vi "view system reservations.vi"(10 "Variant":variant) -> ()   [LabVIEW 2016, in "FPGA Addon System Explorer.lvlib"]
uses:
  FPGA Addon System Explorer.lvlib
  <vilib>/NI VeriStand/Custom Device API/Custom Device API.lvlib
panel:
  in  "Tree":string(tree)
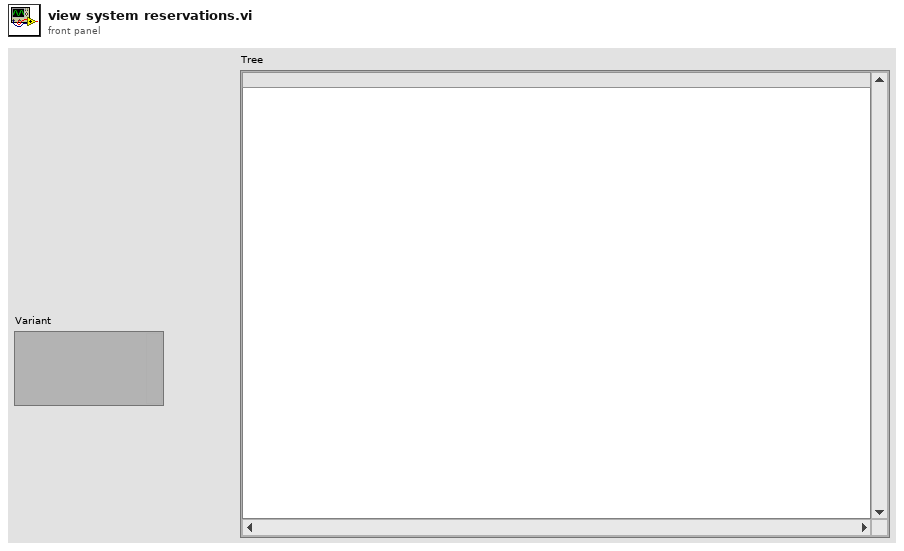
[diagram p1: front panel]
types:
  T1 = typedef "Custom Device API.lvlib/Custom Device Item Info.ctl" = cluster{"Name":string, "Is Channel":bool, "GUID":string, "Is Waveform":bool}
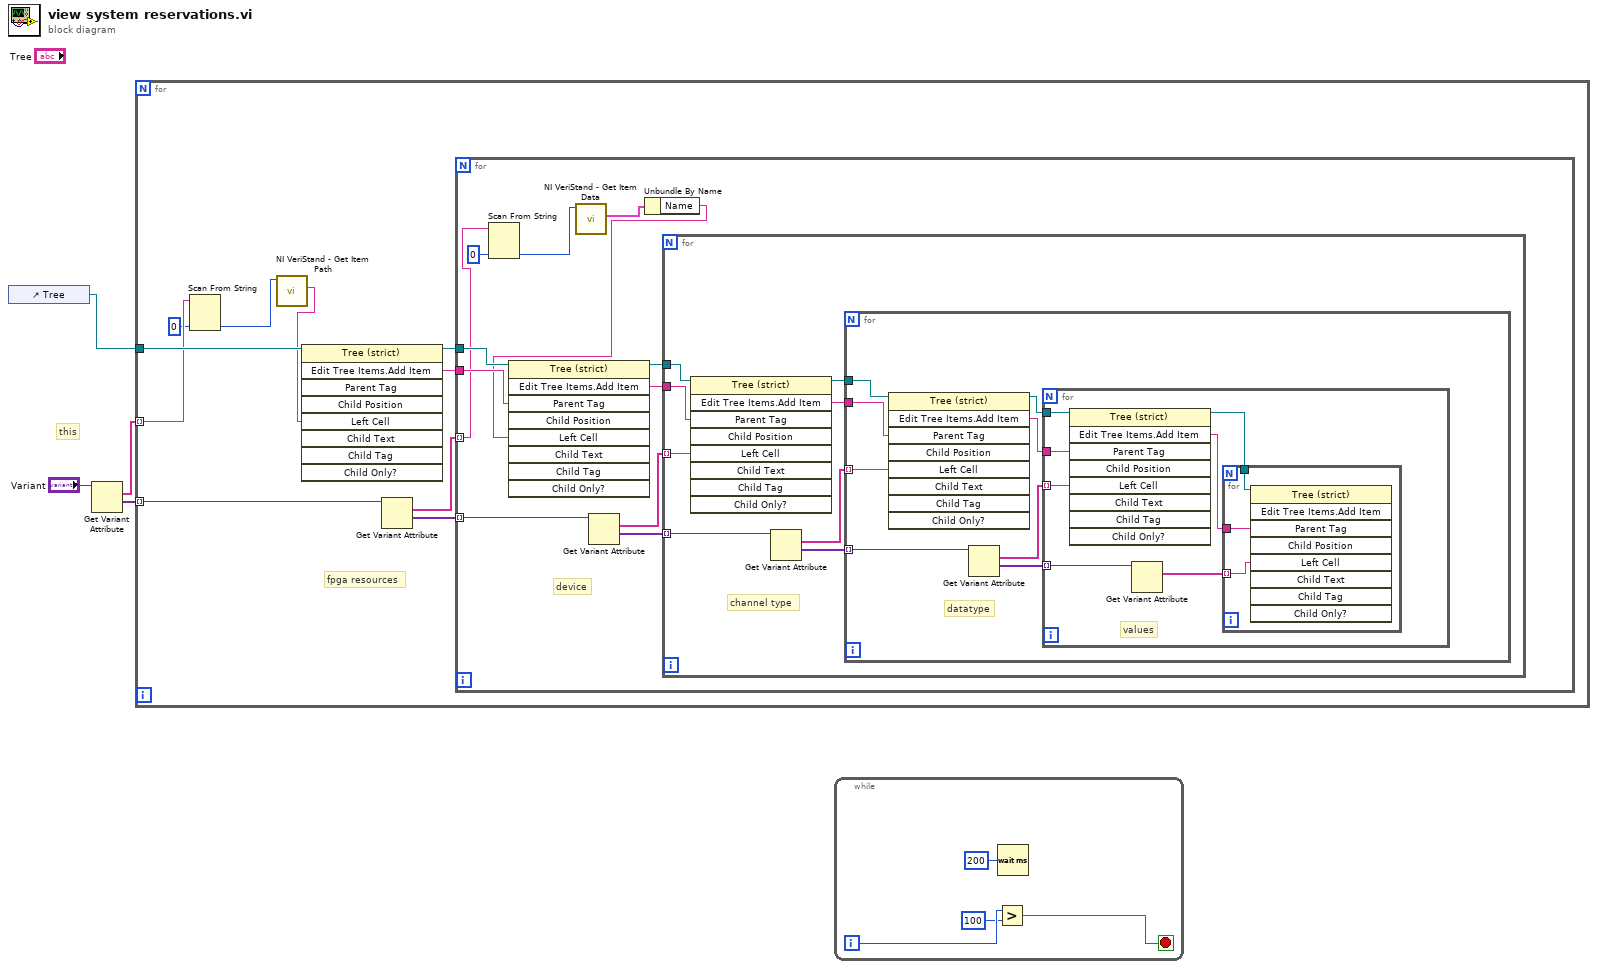
[diagram p0: block diagram]
diagram:
  # "this"
  n1 = control-ref of="Tree"() -> (w1:refnum<vi>)
  n2 = Get Variant Attribute(Variant="Variant") -> (names=w3:string[], values=w2:variant[])  [unwired: 3 in, 2 out]
  n3 = for {
    tunnel: w3 -> [w8] mode=indexing
    tunnel: w2 -> [w14] mode=indexing
    tunnel: w1 -> [w10]
    # "fpga resources"
    n4 = Scan From String(input string=w8, default 1=u64 0 ("default value 1")) -> (output 1=w6:u64)  [unwired: 3 in, 3 out]
    n5 = call <vilib>:"NI VeriStand - Get Item Path.vi"("Item Ref in"=w6) -> ("Path"=w5:string)  [unwired: 7 in, 3 out]
    n6 = invoke on="Invoke Node" class="Tree (strict)" method="Edit Tree Items.Add Item"(reference=w10, "Left Cell"=w5) -> (reference out=w9:refnum<vi>, "Edit Tree Items:Add Item"=w12:string)  [unwired: 7 in, 7 out]
    n7 = Get Variant Attribute(Variant=w14) -> (names=w13:string[], values=w11:variant[])  [unwired: 3 in, 2 out]
    n8 = for {
      tunnel: w13 -> [w15] mode=indexing
      tunnel: w12 -> [w26]
      tunnel: w11 -> [w24] mode=indexing
      tunnel: w9 -> [w21]
      # "device"
      n9 = Scan From String(input string=w15, default 1=u64 0 ("default value 1")) -> (output 1=w19:u64)  [unwired: 3 in, 3 out]
      n10 = call <vilib>:"NI VeriStand - Get Item Data.vi"("Item Ref in"=w19) -> ("Item Info"=w17:T1)  [unwired: 7 in, 3 out]
      n11 = Get Variant Attribute(Variant=w24) -> (names=w23:string[], values=w22:variant[])  [unwired: 3 in, 2 out]
      n12 = Unbundle By Name(w17) -> ("Name"=w16:string)
      n13 = invoke on="Invoke Node" class="Tree (strict)" method="Edit Tree Items.Add Item"(reference=w21, "Parent Tag"=w26, "Left Cell"=w16) -> (reference out=w20:refnum<vi>, "Edit Tree Items:Add Item"=w25:string)  [unwired: 6 in, 7 out]
      n14 = for {
        tunnel: w23 -> [w33] mode=indexing
        tunnel: w25 -> [w34]
        tunnel: w22 -> [w32] mode=indexing
        tunnel: w20 -> [w28]
        # "channel type"
        n15 = invoke on="Invoke Node" class="Tree (strict)" method="Edit Tree Items.Add Item"(reference=w28, "Parent Tag"=w34, "Left Cell"=w33) -> (reference out=w27:refnum<vi>, "Edit Tree Items:Add Item"=w30:string)  [unwired: 6 in, 7 out]
        n16 = Get Variant Attribute(Variant=w32) -> (names=w31:string[], values=w29:variant[])  [unwired: 3 in, 2 out]
        n17 = for {
          tunnel: w31 -> [w41] mode=indexing
          tunnel: w30 -> [w42]
          tunnel: w29 -> [w39] mode=indexing
          tunnel: w27 -> [w35]
          # "datatype"
          n18 = invoke on="Invoke Node" class="Tree (strict)" method="Edit Tree Items.Add Item"(reference=w35, "Parent Tag"=w42, "Left Cell"=w41) -> (reference out=w36:refnum<vi>, "Edit Tree Items:Add Item"=w40:string)  [unwired: 6 in, 7 out]
          n19 = Get Variant Attribute(Variant=w39) -> (names=w38:string[], values=w37:variant[])  [unwired: 3 in, 2 out]
          n20 = for {
            tunnel: w38 -> [w48] mode=indexing
            tunnel: w40 -> [w49]
            tunnel: w37 -> [w46] mode=indexing
            tunnel: w36 -> [w43]
            # "values"
            n21 = invoke on="Invoke Node" class="Tree (strict)" method="Edit Tree Items.Add Item"(reference=w43, "Parent Tag"=w49, "Left Cell"=w48) -> (reference out=w44:refnum<vi>, "Edit Tree Items:Add Item"=w47:string)  [unwired: 6 in, 7 out]
            n22 = Get Variant Attribute(Variant=w46) -> (names=w45:string[])  [unwired: 3 in, 3 out]
            n23 = for {
              tunnel: w45 -> [w51] mode=indexing
              tunnel: w47 -> [w52]
              tunnel: w44 -> [w50]
              n24 = invoke on="Invoke Node" class="Tree (strict)" method="Edit Tree Items.Add Item"(reference=w50, "Parent Tag"=w52, "Left Cell"=w51) -> ()  [unwired: 6 in, 9 out]
            }
          }
        }
      }
    }
  }
  n25 = while {
    i -> [w55]
    stop <- w53 stop-if-true
    n26 = Greater?(x=w55, y=100) -> (0:w53:bool)
    n27 = Wait (ms)(milliseconds to wait=u32 200) -> ()  [unwired: 1 out]
  }
